vi "LoadTemplateFromXML.vi"(4 "Category Nonlocalized Names":string[](array[string]), 6 "Category Names":string[](array[string]), 7 "Project Version Check? (F)":bool, 10 "Template Source Path":path, 11 "XML String In":string) -> (2 "Valid Template?":bool, 3 "Template Out":refnum<class "MetaDataObj.lvclass">)   [LabVIEW 2016, in "NI_NPW_Loading Project Info.lvlib"]
uses:
  <resource>/dialog/NewProjectWizard/Loading Project Info/NI_NPW_Loading Project Info.lvlib
  <resource>/dialog/NewProjectWizard/MetaDataObj/MetaDataObj.lvclass
  <resource>/dialog/NewProjectWizard/MetaDataObj/Accessors/CustomVIModes.ctl
  <resource>/dialog/NewProjectWizard/MetaDataObj/MetaDataObj.lvclass/MetaDataObj.ctl
  <resource>/dialog/NewProjectWizard/MetaDataObj/Accessors/Write Child Class Path.vi
  <resource>/dialog/NewProjectWizard/MetaDataObj/Accessors/Write Panels Minimized.vi
  <resource>/dialog/NewProjectWizard/MetaDataObj/Accessors/Write Panels Open.vi
  <resource>/dialog/NewProjectWizard/MetaDataObj/Accessors/Write Label Localizations.vi
  <resource>/dialog/NewProjectWizard/MetaDataObj/Accessors/Write LocationPath.vi
  <resource>/dialog/NewProjectWizard/MetaDataObj/Accessors/Write Custom VI Mode.vi
  <resource>/dialog/NewProjectWizard/MetaDataObj/Accessors/Write Custom VI Path.vi
  <resource>/dialog/NewProjectWizard/MetaDataObj/Accessors/Write Description.vi
  <resource>/dialog/NewProjectWizard/MetaDataObj/Accessors/Write Documentation Path.vi
  <resource>/dialog/NewProjectWizard/MetaDataObj/Accessors/Write Icon Path.vi
  <resource>/dialog/NewProjectWizard/MetaDataObj/Accessors/Write Icon.vi
  <resource>/dialog/NewProjectWizard/MetaDataObj/Accessors/Write Keywords.vi
  <resource>/dialog/NewProjectWizard/MetaDataObj/Accessors/Write Project Path.vi
  <resource>/dialog/NewProjectWizard/MetaDataObj/Accessors/Write Title.vi
  <resource>/dialog/NewProjectWizard/MetaDataObj/Accessors/Write Filters.vi
  <resource>/dialog/NewProjectWizard/MetaDataObj/Accessors/Write Modes.vi
  <resource>/dialog/NewProjectWizard/MetaDataObj/Accessors/Write Sort Priority.vi
  <resource>/dialog/NewProjectWizard/MetaDataObj/Accessors/Write Version.vi
  <resource>/dialog/NewProjectWizard/MetaDataObj/Accessors/Write Error Codes VI.vi
  <resource>/dialog/NewProjectWizard/MetaDataObj/Accessors/Write Hide Prefix.vi
  <resource>/dialog/NewProjectWizard/MetaDataObj/Accessors/Write Hide Icon Overlay.vi
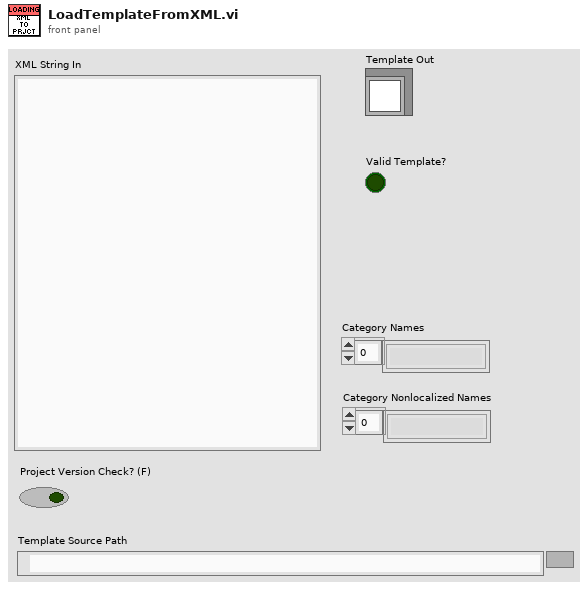
[diagram p1: front panel]
types:
  T1 = typedef "CustomVIModes.ctl" = enum16{"None", "AfterPage1", "AfterPage2WithUI", "AfterPage2NoUI"}
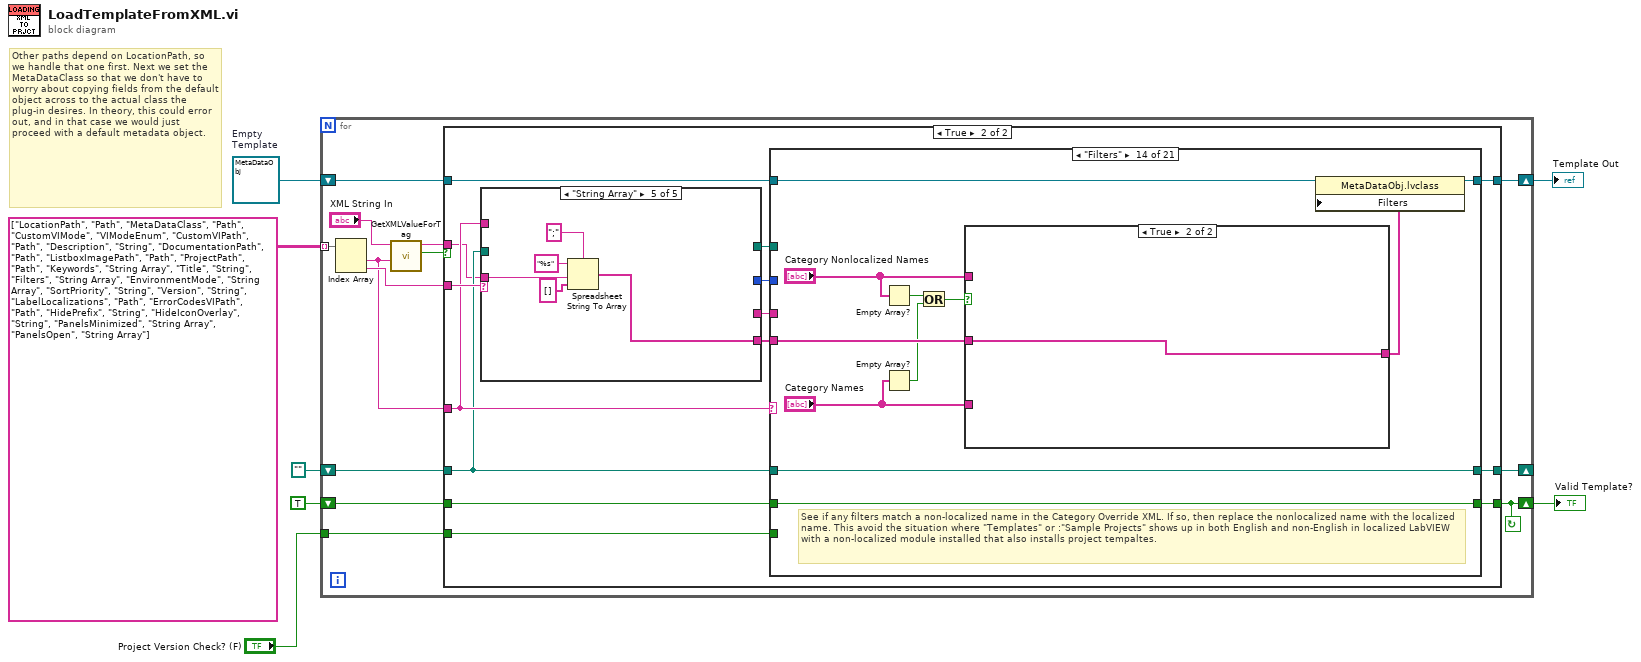
[diagram p0: block diagram]
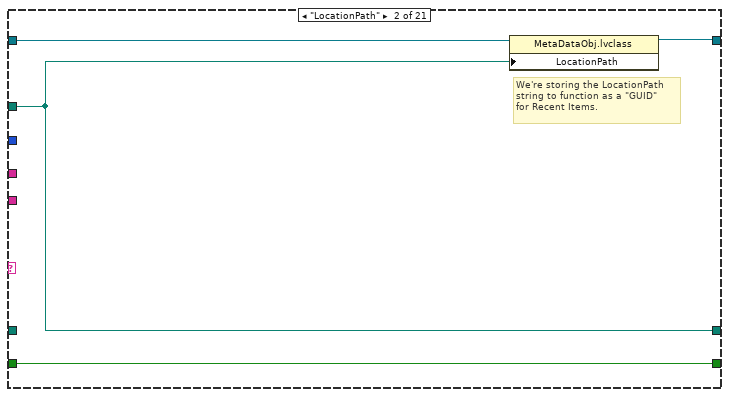
[diagram p4: hidden frame]
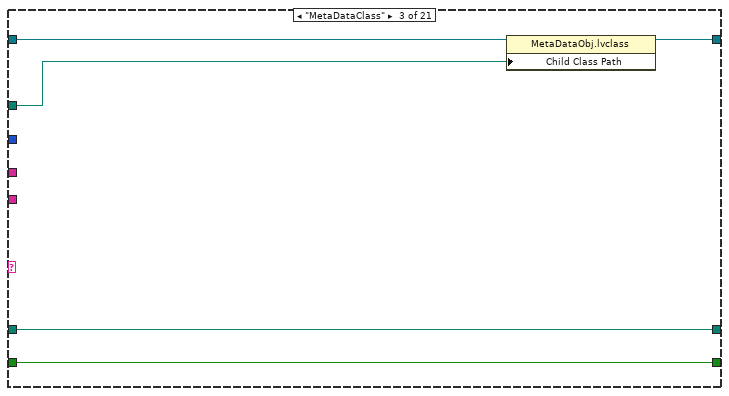
[diagram p5: hidden frame]
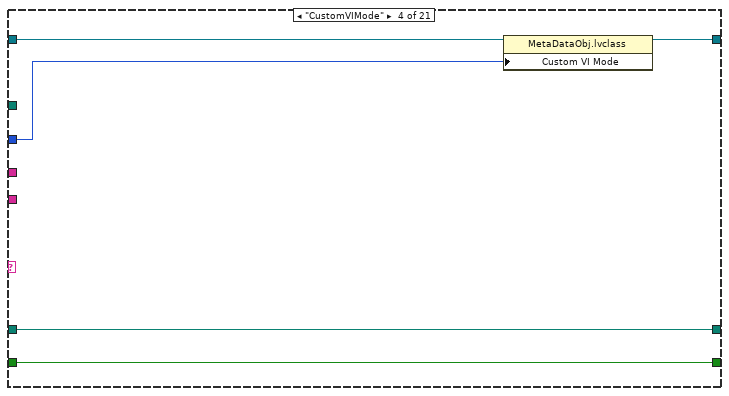
[diagram p6: hidden frame]
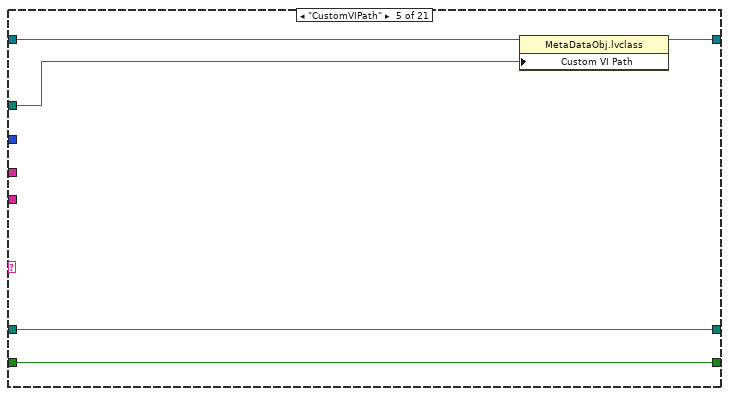
[diagram p7: hidden frame]
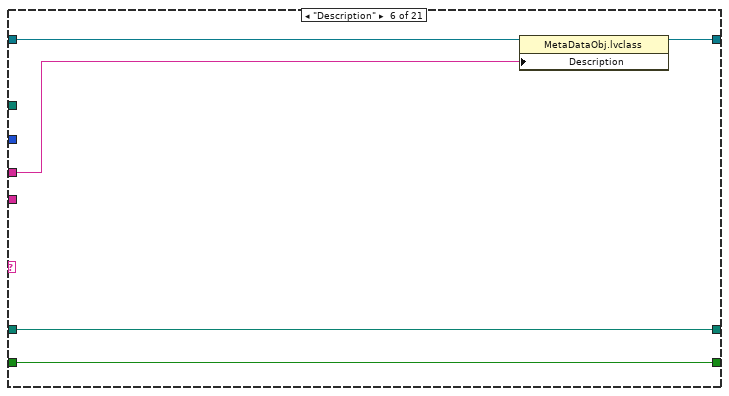
[diagram p8: hidden frame]
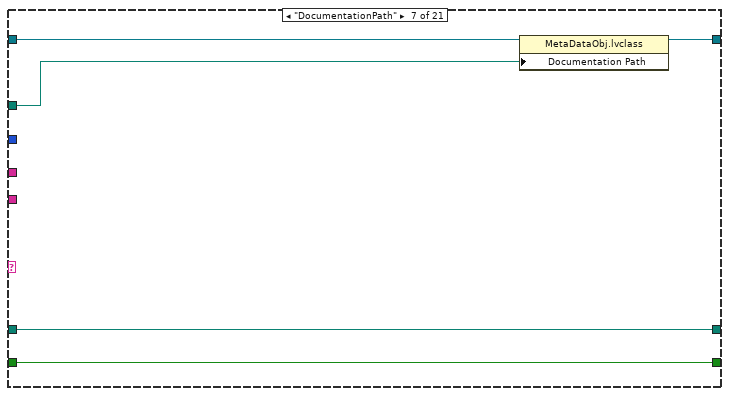
[diagram p9: hidden frame]
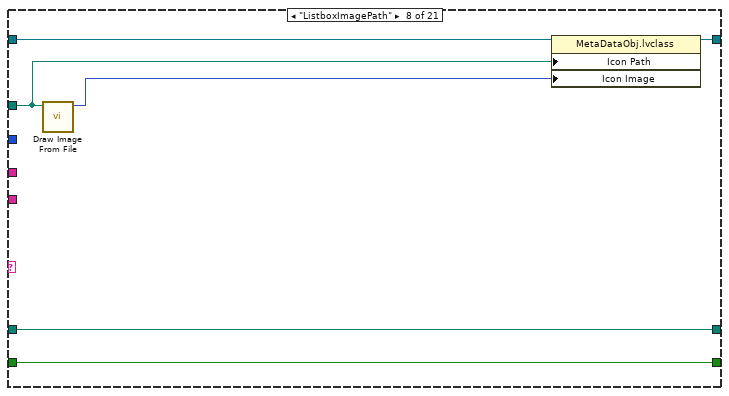
[diagram p10: hidden frame]
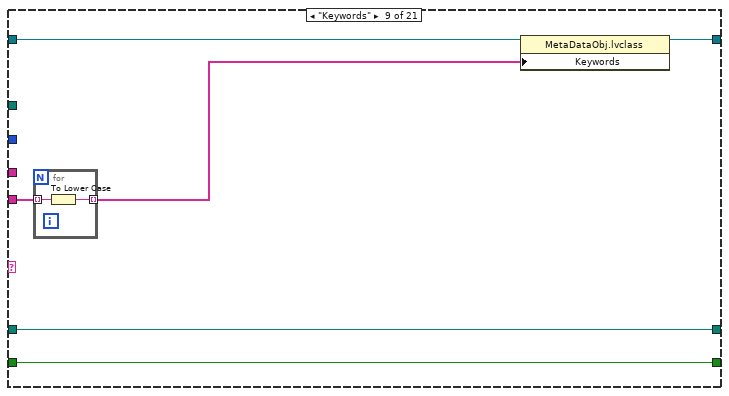
[diagram p11: hidden frame]
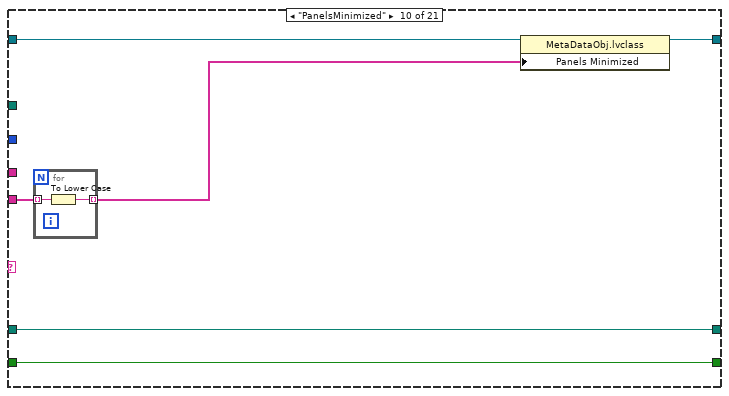
[diagram p12: hidden frame]
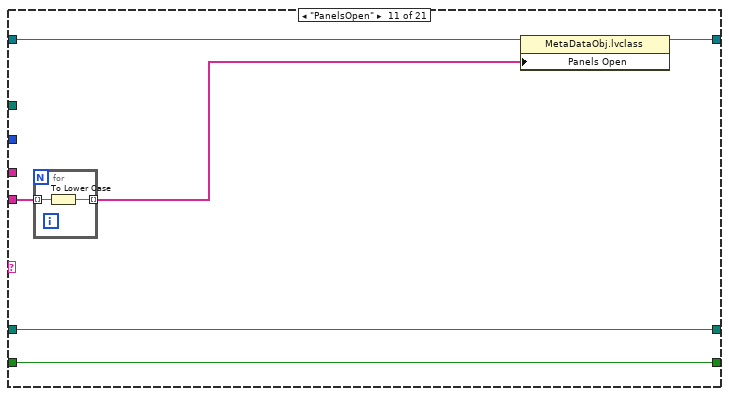
[diagram p13: hidden frame]
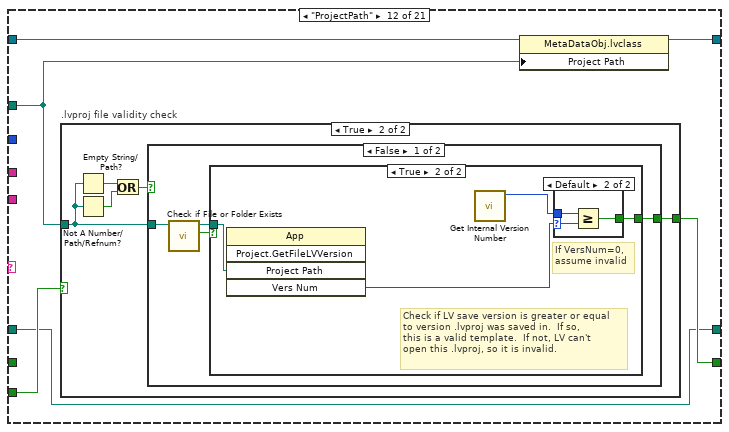
[diagram p14: hidden frame]
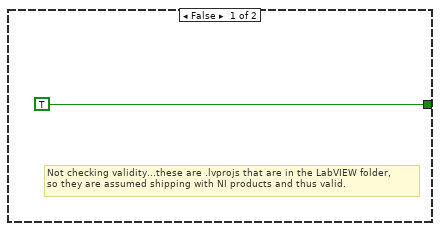
[diagram p15: hidden frame]
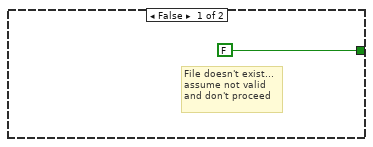
[diagram p16: hidden frame]
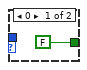
[diagram p17: hidden frame]
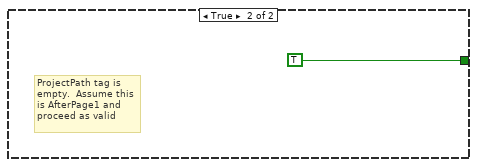
[diagram p18: hidden frame]
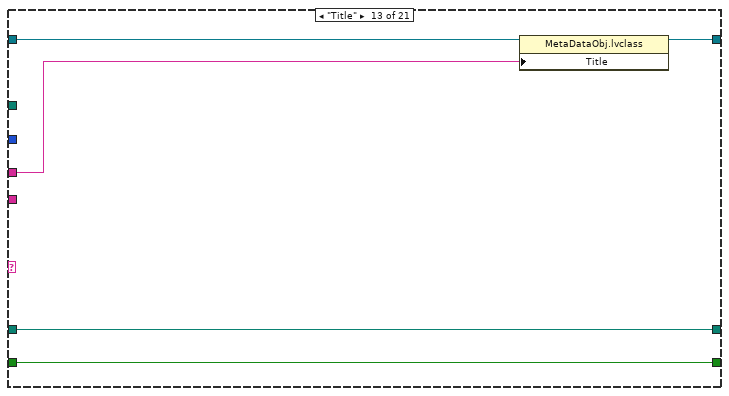
[diagram p19: hidden frame]
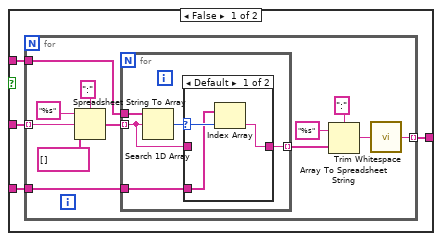
[diagram p20: hidden frame]
diagram:
  w5 = refnum<class "MetaDataObj.lvclass"> refnum  # Empty Template
  # "Other paths depend on LocationPath, so we handle that one first. Next we set the MetaDataClass so that we don't have to worry about copying fields from the default object across to the actual class the plug-in desires. In theory, this could error out, and in that case we would just proceed with a default metadata object."
  n1 = for {
    tunnel: string[][] [["LocationPath", "Path"], ["MetaDataClass", "Path"], ["CustomVIMode", "VIModeEnum"], ["CustomVIPath", "Path"], ["Description", "String"], ["DocumentationPath", "Path"], ["ListboxImagePath", "Path"], ["ProjectPath", "Path"], ["Keywords", "String Array"], ["Title", "String"], ["Filters", "String Array"], ["EnvironmentMode", "String Array"], ["SortPriority", "String"], ["Version", "String"], ["LabelLocalizations", "Path"], ["ErrorCodesVIPath", "Path"], ["HidePrefix", "String"], ["HideIconOverlay", "String"], ["PanelsMinimized", "String Array"], ["PanelsOpen", "String Array"]] -> [w20] mode=indexing
    shift-right: [w16] -> w6
    shift-left: w5 -> [w17]
    shift-right: [w11] -> _
    shift-left: path "" -> [w12]
    shift-right: [w8] -> w2
    shift-left: TRUE -> [w10]
    tunnel: "Project Version Check? (F)" -> [w9]
    stop <- w8 continue-if-true
    n2 = Index Array(array=w20) -> (element #1=w14:string, element #2=w19:string)  [unwired: 2 in]
    n3 = call <resource>:"GetXMLValueForTag.vi"("tag"=w14, "XML"="XML String In") -> ("Found?"=w13:bool, "value"=w18:string)  [unwired: 7 in, 1 out]
    n4 = case shown="True" w13 {
      tunnel: w19 -> [_ w37]
      tunnel: w18 -> [_ w24]
      tunnel: w17 -> [w23 w36]
      tunnel: [w23 w35] -> w16
      tunnel: w14 -> [_ w30]
      tunnel: w12 -> [w22 w28]
      tunnel: [w22 w29] -> w11
      tunnel: w10 -> [w21 w27]
      tunnel: [w21 w26] -> w8
      tunnel: w9 -> [_ w25]
      frame False {
      }
      frame True {
        n5 = case shown="\"String Array\"" w37 {
          tunnel: w24 -> [_ w220 w224 w230 w232]
          tunnel: [_ w219 _ _ _] -> w34
          tunnel: [_ _ w225 _ _] -> w33
          tunnel: [_ _ _ w230 _] -> w31
          tunnel: [_ _ _ _ w231] -> w32
          tunnel: w30 -> [_ _ w227 _ _]
          tunnel: w28 -> [_ _ w223 _ _]
          frame Default {
          }
          frame "VIModeEnum" {
            n6 = Scan From String(format string="%s", input string=w220, default 1=CustomVIModes."None" ("Custom VI Mode")) -> (error out=w218:errorcluster, output 1=w219:T1)  [unwired: 2 in, 2 out]
            n7 = stacked-sequence {
              tunnel: w218 -> [_]
              frame #0 {
                # "Ignore error and just use default."
              }
            }
          }
          frame "Path" {
            n8 = case shown="Default" w227 {
              tunnel: ["Template Source Path" w229] -> w226
              tunnel: w223 -> [_ w229]
              frame "LocationPath" {
              }
              frame Default {
              }
            }
            n9 = call <resource>:"AddStringToPath.vi"("String"=w224, "Path In"=w226) -> ("Path Out"=w225:path)  [unwired: 9 in]
          }
          frame "String" {
          }
          frame "String Array" {
            n10 = Spreadsheet String To Array(delimiter (Tab)=";", format string="%s", spreadsheet string=w232, array type (2D Dbl)=string[] []) -> (array=w231:string[])
          }
        }
        n11 = case shown="\"Filters\"" w30 {
          tunnel: w36 -> [w40 w44 w48 w54 w59 w64 w69 w75 w81 w89 w97 w105 w130 w141 w172 w178 w187 w196 w201 w209 w217]
          tunnel: [w40 w43 w49 w53 w58 w63 w68 w74 w80 w88 w96 w104 w129 w140 w171 w177 w186 w195 w200 w208 w216] -> w35
          tunnel: w34 -> [_ _ _ w52 _ _ _ _ _ _ _ _ _ _ _ _ _ _ _ _ _]
          tunnel: w33 -> [_ w42 w47 _ w57 _ w67 w72 _ _ _ w101 _ _ _ _ _ w194 w199 _ _]
          tunnel: w32 -> [_ _ _ _ _ _ _ _ w79 w87 w95 _ _ w137 w170 _ _ _ _ _ _]
          tunnel: w31 -> [_ _ _ _ _ w62 _ _ _ _ _ _ w128 _ _ w175 w184 _ _ w206 w214]
          tunnel: w28 -> [w39 _ w46 w51 w56 w61 w66 w73 w77 w85 w93 w100 w127 w139 w169 w174 w183 w193 w198 w207 w215]
          tunnel: [w39 w42 w46 w51 w56 w61 w66 w73 w77 w85 w93 w100 w127 w139 w169 w174 w183 w193 w198 w207 w215] -> w29
          tunnel: w27 -> [w38 w41 w45 w50 w55 w60 w65 w70 w76 w84 w92 _ w126 w138 w168 w173 w182 w192 w197 w202 w210]
          tunnel: [w38 w41 w45 w50 w55 w60 w65 w70 w76 w84 w92 w102 w126 w138 w168 w173 w182 w192 w197 w202 w210] -> w26
          tunnel: w25 -> [_ _ _ _ _ _ _ _ _ _ _ w103 _ _ _ _ _ _ _ _ _]
          frame Default {
          }
          frame "LocationPath" {
            # "We're storing the LocationPath\nstring to function as a \"GUID\"\nfor Recent Items."
            n12 = property class="MetaDataObj.lvclass"(reference=w44, "LocationPath"=w42) -> (reference out=w43:refnum<class "MetaDataObj.lvclass">)  [unwired: 1 in, 1 out]
          }
          frame "MetaDataClass" {
            n13 = property class="MetaDataObj.lvclass"(reference=w48, "Child Class Path"=w47) -> (reference out=w49:refnum<class "MetaDataObj.lvclass">)  [unwired: 1 in, 1 out]
          }
          frame "CustomVIMode" {
            n14 = property on="Property Node" class="MetaDataObj.lvclass"(reference=w54, "Custom VI Mode"=w52) -> (reference out=w53:refnum<class "MetaDataObj.lvclass">)  [unwired: 1 in, 1 out]
          }
          frame "CustomVIPath" {
            n15 = property on="Property Node" class="MetaDataObj.lvclass"(reference=w59, "Custom VI Path"=w57) -> (reference out=w58:refnum<class "MetaDataObj.lvclass">)  [unwired: 1 in, 1 out]
          }
          frame "Description" {
            n16 = property on="Property Node" class="MetaDataObj.lvclass"(reference=w64, "Description"=w62) -> (reference out=w63:refnum<class "MetaDataObj.lvclass">)  [unwired: 1 in, 1 out]
          }
          frame "DocumentationPath" {
            n17 = property on="Property Node" class="MetaDataObj.lvclass"(reference=w69, "Documentation Path"=w67) -> (reference out=w68:refnum<class "MetaDataObj.lvclass">)  [unwired: 1 in, 1 out]
          }
          frame "ListboxImagePath" {
            n18 = call <resource>:"Draw Image From File.vi"("Image Path In"=w72) -> ("Picture Out"=w71:picture)  [unwired: 9 in, 1 out]
            n19 = property on="Property Node" class="MetaDataObj.lvclass"(reference=w75, "Icon Path"=w72, "Icon Image"=w71) -> (reference out=w74:refnum<class "MetaDataObj.lvclass">)  [unwired: 1 in, 1 out]
          }
          frame "Keywords" {
            n20 = for {
              tunnel: w79 -> [w83] mode=indexing
              tunnel: [w82] -> w78 mode=indexing
              n21 = To Lower Case(string=w83) -> (all lower case string=w82:string)
            }
            n22 = property on="Property Node" class="MetaDataObj.lvclass"(reference=w81, "Keywords"=w78) -> (reference out=w80:refnum<class "MetaDataObj.lvclass">)  [unwired: 1 in, 1 out]
          }
          frame "PanelsMinimized" {
            n23 = for {
              tunnel: w87 -> [w91] mode=indexing
              tunnel: [w90] -> w86 mode=indexing
              n24 = To Lower Case(string=w91) -> (all lower case string=w90:string)
            }
            n25 = property on="Property Node" class="MetaDataObj.lvclass"(reference=w89, "Panels Minimized"=w86) -> (reference out=w88:refnum<class "MetaDataObj.lvclass">)  [unwired: 1 in, 1 out]
          }
          frame "PanelsOpen" {
            n26 = for {
              tunnel: w95 -> [w99] mode=indexing
              tunnel: [w98] -> w94 mode=indexing
              n27 = To Lower Case(string=w99) -> (all lower case string=w98:string)
            }
            n28 = property on="Property Node" class="MetaDataObj.lvclass"(reference=w97, "Panels Open"=w94) -> (reference out=w96:refnum<class "MetaDataObj.lvclass">)  [unwired: 1 in, 1 out]
          }
          frame "ProjectPath" {
            n29 = case ".lvproj file validity check" shown="True" w103 {
              tunnel: [TRUE w108] -> w102
              tunnel: w101 -> [_ w107]
              frame False {
                # "Not checking validity...these are .lvprojs that are in the LabVIEW folder,\nso they are assumed shipping with NI products and thus valid."
              }
              frame True {
                n30 = Empty String/Path?(string/path=w107) -> (empty?=w111:bool)
                n31 = Not A Number/Path/Refnum?(number/path/refnum=w107) -> (NaN/Path/Refnum?=w110:bool)
                n32 = Or(x=w111, y=w110) -> (x .or. y?=w109:bool)
                n33 = case shown="False" w109 {
                  tunnel: [w112 TRUE] -> w108
                  tunnel: w107 -> [w115 _]
                  frame False {
                    n34 = call <vilib>:"Check if File or Folder Exists.vi"("path"=w115) -> ("file or folder exists?"=w114:bool, "dup path"=w113:path)  [unwired: 8 in, 1 out]
                    n35 = case shown="True" w114 {
                      tunnel: w113 -> [_ w120]
                      tunnel: [FALSE w118] -> w112
                      frame False {
                        # "File doesn't exist...\nassume not valid\nand don't proceed"
                      }
                      frame True {
                        # "If VersNum=0,\nassume invalid"
                        # "Check if LV save version is greater or equal\nto version .lvproj was saved in.  If so,\nthis is a valid template.  If not, LV can't\nopen this .lvproj, so it is invalid."
                        n36 = invoke class="App" method="Project.GetFileLVVersion"("Project Path"=w120) -> ("Vers Num"=w117:u32)  [unwired: 4 in, 4 out]
                        n37 = call <resource>:"Get Internal Version Number.vi"() -> ("App.SaveVerLVFmt"=w119:i32)  [unwired: 11 in]
                        n38 = case shown="Default" w117 {
                          selector: w117 -> [_ w122]
                          tunnel: w119 -> [_ w124]
                          tunnel: [FALSE w123] -> w118
                          frame 0 {
                          }
                          frame Default {
                            n39 = Greater Or Equal?(x=w124, y=w122) -> (x >= y?=w123:bool)
                          }
                        }
                      }
                    }
                  }
                  frame True {
                    # "ProjectPath tag is empty.  Assume this is AfterPage1 and proceed as valid"
                  }
                }
              }
            }
            n40 = property on="Property Node" class="MetaDataObj.lvclass"(reference=w105, "Project Path"=w101) -> (reference out=w104:refnum<class "MetaDataObj.lvclass">)  [unwired: 1 in, 1 out]
          }
          frame "Title" {
            n41 = property on="Property Node" class="MetaDataObj.lvclass"(reference=w130, "Title"=w128) -> (reference out=w129:refnum<class "MetaDataObj.lvclass">)  [unwired: 1 in, 1 out]
          }
          frame "Filters" {
            # "See if any filters match a non-localized name in the Category Override XML. If so, then replace the nonlocalized name with the localized name. This avoid the situation where \"Templates\" or :\"Sample Projects\" shows up in both English and non-English in localized LabVIEW with a non-localized module installed that also installs project tempaltes."
            n42 = Empty Array?(array="Category Nonlocalized Names") -> (empty?=w134:bool)
            n43 = Empty Array?(array="Category Names") -> (empty?=w132:bool)
            n44 = Or(x=w134, y=w132) -> (x .or. y?=w131:bool)
            n45 = case shown="True" w131 {
              tunnel: w137 -> [w145 w167]
              tunnel: [w144 w167] -> w136
              tunnel: "Category Nonlocalized Names" -> [w143 _]
              tunnel: "Category Names" -> [w142 _]
              frame False {
                n46 = for {
                  tunnel: w145 -> [w157] mode=indexing
                  tunnel: w143 -> [w152]
                  tunnel: w142 -> [w151]
                  tunnel: [w146] -> w144 mode=indexing
                  n47 = Spreadsheet String To Array(delimiter (Tab)=":", format string="%s", spreadsheet string=w157, array type (2D Dbl)=string[] []) -> (array=w153:string[])
                  n48 = for {
                    tunnel: w153 -> [w160] mode=indexing
                    tunnel: w152 -> [w162]
                    tunnel: w151 -> [w159]
                    tunnel: [w158] -> w150 mode=indexing
                    n49 = Search 1D Array(1D array=w162, element=w160) -> (index of element=w161:i32)  [unwired: 1 in]
                    n50 = case shown="Default" w161 {
                      selector: w161 -> [w165 _]
                      tunnel: w160 -> [_ w166]
                      tunnel: w159 -> [w164 _]
                      tunnel: [w163 w166] -> w158
                      frame Default {
                        n51 = Index Array(array=w164, index=w165) -> (element=w163:string)
                      }
                      frame -1 {
                      }
                    }
                  }
                  n52 = Array To Spreadsheet String(delimiter (Tab)=":", array=w150, 3:"%s" ("format string")) -> (spreadsheet string=w147:string)
                  n53 = call <vilib>:"Trim Whitespace.vi"("string"=w147) -> ("trimmed string"=w146:string)  [unwired: 1 in]
                }
              }
              frame True {
              }
            }
            n54 = property on="Property Node" class="MetaDataObj.lvclass"(reference=w141, "Filters"=w136) -> (reference out=w140:refnum<class "MetaDataObj.lvclass">)  [unwired: 1 in, 1 out]
          }
          frame "EnvironmentMode" {
            n55 = property on="Property Node" class="MetaDataObj.lvclass"(reference=w172, "Modes"=w170) -> (reference out=w171:refnum<class "MetaDataObj.lvclass">)  [unwired: 1 in, 1 out]
          }
          frame "SortPriority" {
            # "Sort Priority is a DBL to always allow us\nto shimmy new templates in between\neach other if we have to"
            n56 = case shown="Default" w175 {
              selector: w175 -> [w179 _]
              tunnel: [w180 w181] -> w176
              frame Default {
                n57 = Fract/Exp String To Number(string=w179) -> (number=w180:dbl)  [unwired: 3 in, 1 out]
              }
              frame "" {
                w181 = 2147483647.0  # Default Value
              }
            }
            n58 = property on="Property Node" class="MetaDataObj.lvclass"(reference=w178, "Sort Priority"=w176) -> (reference out=w177:refnum<class "MetaDataObj.lvclass">)  [unwired: 1 in, 1 out]
          }
          frame "Version" {
            n59 = case shown="Default" w184 {
              tunnel: w184 -> [w190 _]
              tunnel: [w189 w191] -> w185
              frame Default {
                n60 = Decimal String To Number(string=w190, default (0L)=u8 0 ("Default Value")) -> (number=w189:u8)  [unwired: 1 in, 1 out]
              }
              frame "" {
                w191 = u8 0  # Default Value
              }
            }
            n61 = property on="Property Node" class="MetaDataObj.lvclass"(reference=w187, "Version"=w185) -> (reference out=w186:refnum<class "MetaDataObj.lvclass">)  [unwired: 1 in, 1 out]
          }
          frame "LabelLocalizations" {
            n62 = property class="MetaDataObj.lvclass"(reference=w196, "Label Localizations"=w194) -> (reference out=w195:refnum<class "MetaDataObj.lvclass">)  [unwired: 1 in, 1 out]
          }
          frame "ErrorCodesVIPath" {
            n63 = property class="MetaDataObj.lvclass"(reference=w201, "Error Codes VI"=w199) -> (reference out=w200:refnum<class "MetaDataObj.lvclass">)  [unwired: 1 in, 1 out]
          }
          frame "HidePrefix" {
            n64 = To Lower Case(string=w206) -> (all lower case string=w205:string)
            n65 = Equal?(x="true", y=w205) -> (x = y?=w203:bool)
            n66 = property class="MetaDataObj.lvclass"(reference=w209, "Hide Prefix?"=w203) -> (reference out=w208:refnum<class "MetaDataObj.lvclass">)  [unwired: 1 in, 1 out]
          }
          frame "HideIconOverlay" {
            n67 = To Lower Case(string=w214) -> (all lower case string=w213:string)
            n68 = Equal?(x="true", y=w213) -> (x = y?=w211:bool)
            n69 = property class="MetaDataObj.lvclass"(reference=w217, "Hide Icon Overlay?"=w211) -> (reference out=w216:refnum<class "MetaDataObj.lvclass">)  [unwired: 1 in, 1 out]
          }
        }
      }
    }
  }
  "Template Out" <- w6
  "Valid Template?" <- w2
